vi "Set__slk_mt.vi"(7 "values":string[][](array[string]), 8 "error in (no error)":errorcluster, 11 "combobox in":refnum<class "ComboBox__slk_mt.lvclass">) -> (0 "error out":errorcluster, 3 "combobox out":refnum<class "ComboBox__slk_mt.lvclass">)   [LabVIEW 2020, in "ComboBox__slk_mt.lvclass"]
doc: "Sets the values to the control on GUI.\n\n<b>Values:</b>\n[ [Section, Key, Value], [Section, Key, Value], ..., [Section, Key, Value] ]"
uses:
  ComboBox__slk_mt.lvclass
  ComboBox__slk_mt.lvclass/ComboBox__slk_mt.ctl
panel:
  # "Set__slk_mt.vi\nSets the values to the control on GUI.\n\nNOTICE -- YOU MUST LEAVE THIS NOTICE IN PLACE.\n\nCopyright (c) 2011, LIANG LIU Shawn.Liu.cn@gmail.com\nAll rights reserved.\n\nRedistribution and use in source and binary forms, with or without modification, are permitted provided that the following conditions are met:\n-Redistributions of source code must retain the above copyright notice, this list of conditions and the following disclaimer.\n-Redistributions in binary form must reproduce the above copyright notice, this list of conditions and the following disclaimer in the documentation and/or other materials provided with the distribution.\n-Neither the name of the eLp nor the names of its contributors may be used to endorse or promote products derived from this software without specific prior written permission.\n\nTHIS SOFTWARE IS PROVIDED BY THE COPYRIGHT HOLDERS AND CONTRIBUTORS \"AS IS\" AND ANY EXPRESS OR IMPLIED WARRANTIES, INCLUDING, BUT NOT LIMITED TO, THE IMPLIED WARRANTIES OF MERCHANTABILITY AND FITNESS FOR A PARTICULAR PURPOSE ARE DISCLAIMED. IN NO EVENT SHALL THE COPYRIGHT HOLDER OR CONTRIBUTORS BE LIABLE FOR ANY DIRECT, INDIRECT, INCIDENTAL, SPECIAL, EXEMPLARY, OR CONSEQUENTIAL DAMAGES (INCLUDING, BUT NOT LIMITED TO, PROCUREMENT OF SUBSTITUTE GOODS OR SERVICES; LOSS OF USE, DATA, OR PROFITS; OR BUSINESS INTERRUPTION) HOWEVER CAUSED AND ON ANY THEORY OF LIABILITY, WHETHER IN CONTRACT, STRICT LIABILITY, OR TORT (INCLUDING NEGLIGENCE OR OTHERWISE) ARISING IN ANY WAY OUT OF THE USE OF THIS SOFTWARE, EVEN IF ADVISED OF THE POSSIBILITY OF SUCH DAMAGE."
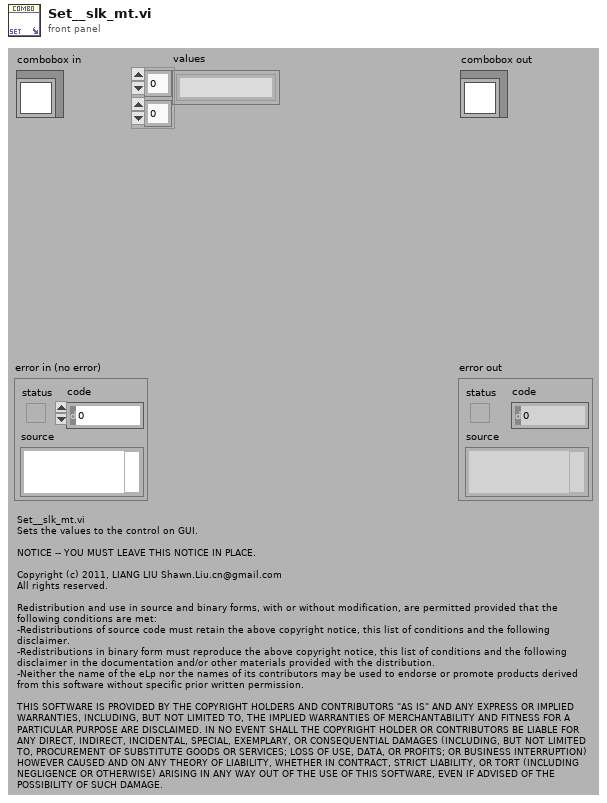
[diagram p1: front panel]
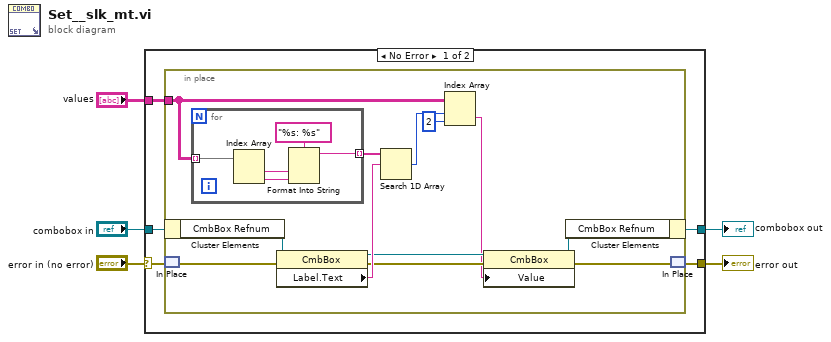
[diagram p0: block diagram]
diagram:
  n1 = case shown="No Error" "error in (no error)" {
    selector: "error in (no error)" -> [w7 w29]
    tunnel: "values" -> [w10 _]
    tunnel: "combobox in" -> [w9 w28]
    tunnel: [w8 w28] -> w3
    tunnel: [w6 w29] -> w1
    frame No Error {
      n2 = in-place {
        in-place-border: w10 -> [w15]
        n3 = in-place-cluster #1(w9) -> ("CmbBox Refnum"=w14:refnum<vi>)
        n4 = in-place-match #2(w7) -> (w12:errorcluster)
        n5 = for {
          tunnel: w15 -> [w27] mode=indexing
          tunnel: [w23] -> w22 mode=indexing
          n6 = Index Array(array=w27) -> (element #1=w25:string, element #2=w24:string)  [unwired: 2 in]
          n7 = Format Into String(format string="%s: %s", w25, w24) -> (resulting string=w23:string)  [unwired: 2 in, 1 out]
        }
        n8 = property class="CmbBox"(reference=w14, error in=w12) -> (reference out=w17:refnum<vi>, error out=w18:errorcluster, "Label.Text"=w19:string)
        n9 = Search 1D Array(1D array=w22, element=w19) -> (index of element=w20:i32)  [unwired: 1 in]
        n10 = Index Array(array=w15, index (row)=w20, index (col)=2 ("disabled index (col)")) -> (element=w16:string)
        n11 = property class="CmbBox"(reference=w17, error in=w18, "Value"=w16) -> (reference out=w13:refnum<vi>, error out=w11:errorcluster)
        n12 = in-place-cluster #1("CmbBox Refnum"=w13) -> (w8:refnum<class "ComboBox__slk_mt.lvclass">)
        n13 = in-place-match #2(w11) -> (w6:errorcluster)
      }
    }
    frame Error {
    }
  }
  "error out" <- w1
  "combobox out" <- w3
